vi "Find True Values in Array.vi"(1 "Mask":bool[](array[boolean])) -> (0 "Indices":i32[](array[numeric]))   [LabVIEW 2015]
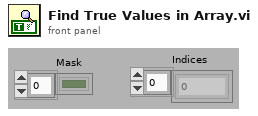
[diagram p1: front panel]
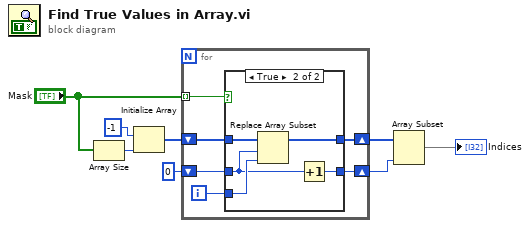
[diagram p0: block diagram]
diagram:
  n1 = Array Size(array="Mask") -> (size(s)=w8:i32)
  n2 = Initialize Array(-1, w8) -> (w5:i32[])
  n3 = for {
    tunnel: "Mask" -> [w14] mode=indexing
    shift-right: [w10] -> w3
    shift-left: w5 -> [w13]
    shift-right: [w9] -> w1
    shift-left: 0 -> [w11]
    i -> [w12]
    n4 = case shown="True" w14 {
      tunnel: w13 -> [w16 w21]
      tunnel: w12 -> [_ w20]
      tunnel: w11 -> [w15 w18]
      tunnel: [w15 w17] -> w9
      tunnel: [w16 w19] -> w10
      frame False {
      }
      frame True {
        n5 = Replace Array Subset(array=w21, new element=w20, index=w18) -> (w19:i32[])
        n6 = Increment(x=w18) -> (x+1=w17:i32)
      }
    }
  }
  n7 = Array Subset(array=w3, length=w1) -> (→"Indices":i32[])  [unwired: 1 in]
